vi "SeCrTs-CDT DIVIDER.vi"(7 "Enum":enum16{"SEQ", "CDT"}(ring), 11 "Seq in":T1(array[cluster])) -> (3 "Array":T2(array[cluster]))   [LabVIEW 2022 SP3]
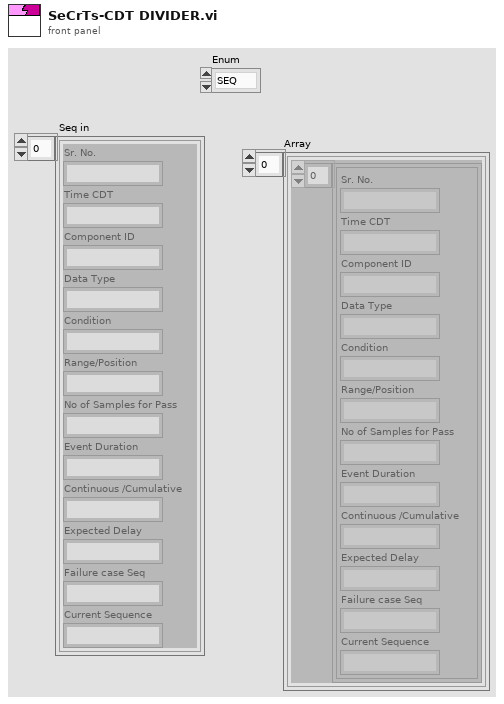
[diagram p1: front panel]
types:
  T1 = cluster{"Sr. No.":string, "Time CDT":string, "Component ID":string, "Data Type":string, "Condition":string, "Range/Position":string, "No of Samples for Pass":string, "Event Duration":string, "Continuous /Cumulative":string, "Expected Delay":string, "Failure case Seq":string, "Current Sequence":string}[]
  T2 = cluster{cluster{"Sr. No.":string, "Time CDT":string, "Component ID":string, "Data Type":string, "Condition":string, "Range/Position":string, "No of Samples for Pass":string, "Event Duration":string, "Continuous /Cumulative":string, "Expected Delay":string, "Failure case Seq":string, "Current Sequence":string}[]}[]
  T3 = cluster{"Sr. No.":string, "Time CDT":string, "Component ID":string, "Data Type":string, "Condition":string, "Range/Position":string, "No of Samples for Pass":string, "Event Duration":string, "Continuous /Cumulative":string, "Expected Delay":string, "Failure case Seq":string, "Current Sequence":string}
  T4 = cluster{cluster{"Sr. No.":string, "Time CDT":string, "Component ID":string, "Data Type":string, "Condition":string, "Range/Position":string, "No of Samples for Pass":string, "Event Duration":string, "Continuous /Cumulative":string, "Expected Delay":string, "Failure case Seq":string, "Current Sequence":string}[]}
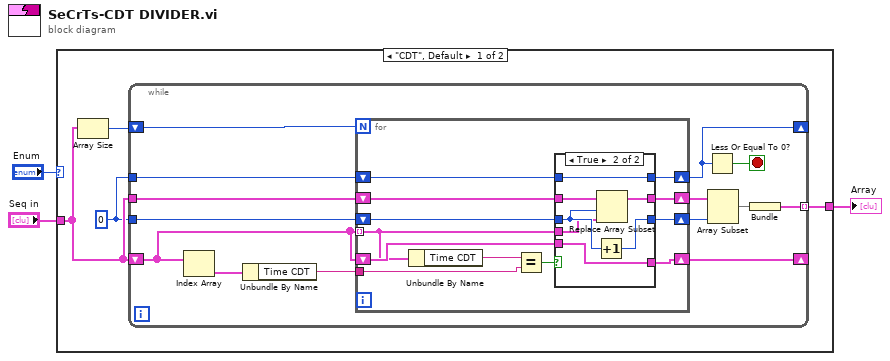
[diagram p0: block diagram]
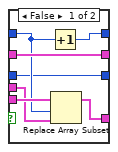
[diagram p2: hidden frame]
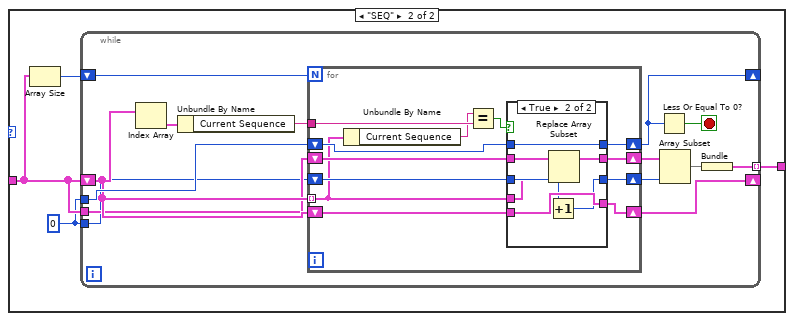
[diagram p3: hidden frame]
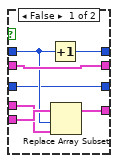
[diagram p4: hidden frame]
diagram:
  n1 = case shown="\"CDT\", Default" "Enum" {
    tunnel: [w7 w51] -> w1
    tunnel: "Seq in" -> [w6 w50]
    frame "CDT", Default {
      w4 = 0 ("index")
      n2 = Array Size(array=w6) -> (size(s)=w5:i32)
      n3 = while {
        shift-right: [w20] -> _
        shift-left: w6 -> [w14]
        tunnel: w4 -> [w21]
        tunnel: [w19] -> w7 mode=indexing
        shift-right: [w16] -> _
        shift-left: w5 -> [w17]
        tunnel: w6 -> [w13]
        tunnel: w4 -> [w12]
        stop <- w15 stop-if-true
        n4 = Index Array(array=w14) -> (element=w18:T3)  [unwired: 1 in]
        n5 = Unbundle By Name(w18) -> ("Time CDT"=w9:string)
        n6 = for {
          N: w17 -> [_]
          shift-right: [w33] -> w20
          shift-left: w14 -> [w30]
          tunnel: w14 -> [w24] mode=indexing
          shift-right: [w32] -> w16
          shift-left: w21 -> [w29]
          shift-right: [w31] -> w11
          shift-left: w13 -> [w28]
          tunnel: w9 -> [w27]
          shift-right: [w25] -> w10
          shift-left: w12 -> [w26]
          n7 = Unbundle By Name(w24) -> ("Time CDT"=w23:string)
          n8 = Equal?(x=w23, y=w27) -> (x = y?=w22:bool)
          n9 = case shown="True" w22 {
            tunnel: w30 -> [w40 w47]
            tunnel: [w39 w47] -> w33
            tunnel: [w38 w46] -> w32
            tunnel: [w37 w43] -> w31
            tunnel: w28 -> [w37 w44]
            tunnel: w29 -> [w36 w46]
            tunnel: w24 -> [w35 w41]
            tunnel: w26 -> [w34 w42]
            tunnel: [w34 w45] -> w25
            frame False {
              n10 = Increment(x=w36) -> (x+1=w38:i32)
              n11 = Replace Array Subset(array=w40, new element=w35, index=w36) -> (w39:T1)
            }
            frame True {
              n12 = Increment(x=w42) -> (x+1=w45:i32)
              n13 = Replace Array Subset(array=w44, new element=w41, index=w42) -> (w43:T1)
            }
          }
        }
        n14 = Less Or Equal To 0?(x=w16) -> (x <= 0?=w15:bool)
        n15 = Array Subset(array=w11, length=w10) -> (w8:T1)  [unwired: 1 in]
        n16 = Bundle(w8) -> (w19:T4)  [unwired: 1 in]
      }
    }
    frame "SEQ" {
      w48 = 0 ("index")
      n17 = Array Size(array=w50) -> (size(s)=w49:i32)
      n18 = while {
        shift-right: [w64] -> _
        shift-left: w50 -> [w58]
        tunnel: w48 -> [w65]
        tunnel: [w63] -> w51 mode=indexing
        shift-right: [w60] -> _
        shift-left: w49 -> [w61]
        tunnel: w50 -> [w57]
        tunnel: w48 -> [w56]
        stop <- w59 stop-if-true
        n19 = Index Array(array=w58) -> (element=w62:T3)  [unwired: 1 in]
        n20 = Unbundle By Name(w62) -> ("Current Sequence"=w53:string)
        n21 = for {
          N: w61 -> [_]
          shift-right: [w77] -> w64
          shift-left: w58 -> [w74]
          tunnel: w58 -> [w68] mode=indexing
          shift-right: [w76] -> w60
          shift-left: w65 -> [w73]
          shift-right: [w75] -> w55
          shift-left: w57 -> [w72]
          tunnel: w53 -> [w71]
          shift-right: [w69] -> w54
          shift-left: w56 -> [w70]
          n22 = Unbundle By Name(w68) -> ("Current Sequence"=w67:string)
          n23 = Equal?(x=w67, y=w71) -> (x = y?=w66:bool)
          n24 = case shown="True" w66 {
            tunnel: w74 -> [w84 w91]
            tunnel: [w83 w91] -> w77
            tunnel: [w82 w90] -> w76
            tunnel: [w81 w87] -> w75
            tunnel: w72 -> [w81 w88]
            tunnel: w73 -> [w80 w90]
            tunnel: w68 -> [w79 w85]
            tunnel: w70 -> [w78 w86]
            tunnel: [w78 w89] -> w69
            frame False {
              n25 = Increment(x=w80) -> (x+1=w82:i32)
              n26 = Replace Array Subset(array=w84, new element=w79, index=w80) -> (w83:T1)
            }
            frame True {
              n27 = Increment(x=w86) -> (x+1=w89:i32)
              n28 = Replace Array Subset(array=w88, new element=w85, index=w86) -> (w87:T1)
            }
          }
        }
        n29 = Less Or Equal To 0?(x=w60) -> (x <= 0?=w59:bool)
        n30 = Array Subset(array=w55, length=w54) -> (w52:T1)  [unwired: 1 in]
        n31 = Bundle(w52) -> (w63:T4)  [unwired: 1 in]
      }
    }
  }
  "Array" <- w1
